vi "ConfigPort.vi"() -> ()   [LabVIEW 2017]
panel:
  in  "退出":bool
  in  "保存":bool
  in  "配置信息":i32(listbox)
  # "多通道连接端口配置"
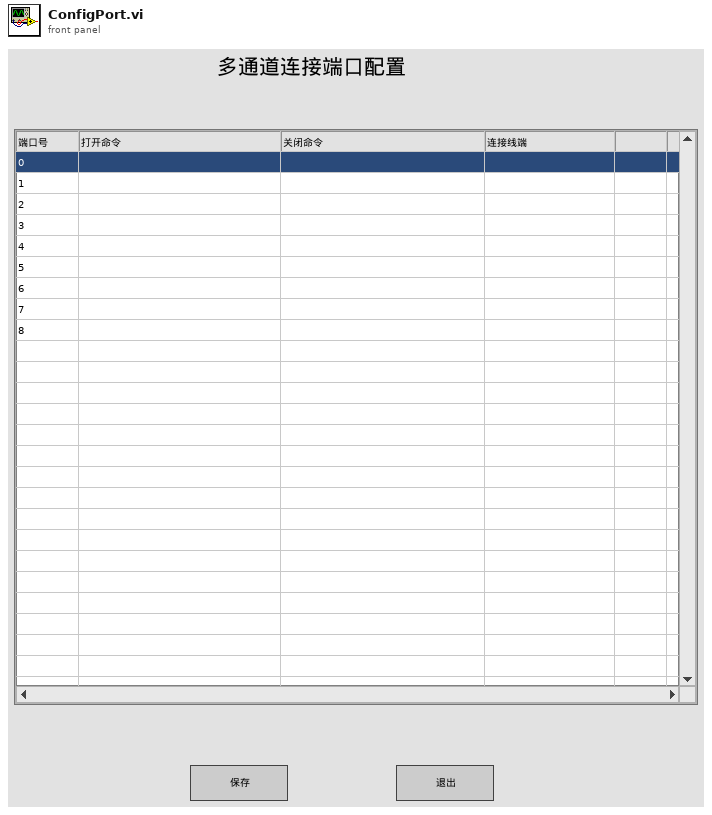
[diagram p1: front panel]
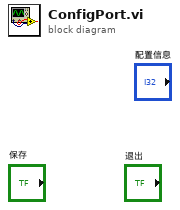
[diagram p0: block diagram]
diagram:
